vi "login.vi"(8 "error in (no error)":errorcluster, 10 "element":string, 11 "Masterv2 in":refnum<class "Masterv2.lvclass">) -> (0 "error out":errorcluster, 2 "x >= 0?":bool, 3 "Masterv2 out":refnum<class "Masterv2.lvclass">)   [LabVIEW 2014, in "Main Libraryv2.lvlib" / "Masterv2.lvclass"]
uses:
  Master/Masterv2.lvclass
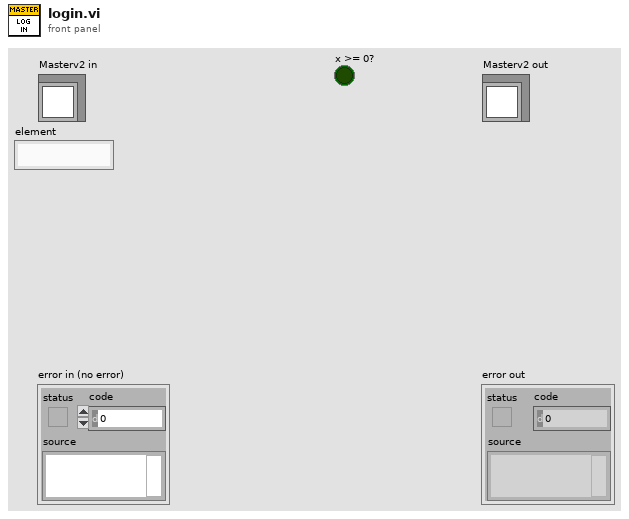
[diagram p1: front panel]
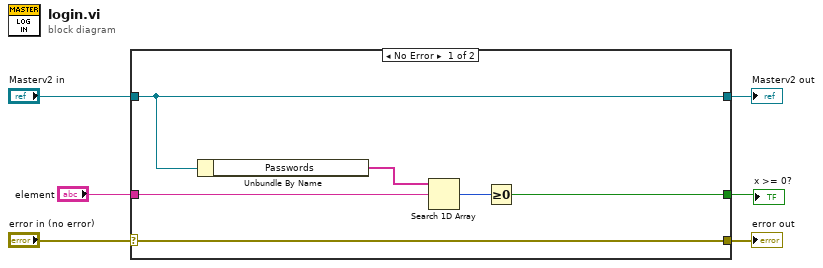
[diagram p0: block diagram]
diagram:
  n1 = case shown="No Error" "error in (no error)" {
    selector: "error in (no error)" -> [w7 w14]
    tunnel: [w7 w14] -> w5
    tunnel: [w8 w13] -> w3
    tunnel: "Masterv2 in" -> [w8 w13]
    tunnel: [w10 _] -> w2
    tunnel: "element" -> [w9 _]
    frame No Error {
      n2 = Unbundle By Name(w8) -> ("Passwords"=w12:string[])
      n3 = Search 1D Array(1D array=w12, element=w9) -> (index of element=w11:i32)  [unwired: 1 in]
      n4 = Greater Or Equal To 0?(x=w11) -> (x >= 0?=w10:bool)
    }
    frame Error {
    }
  }
  "error out" <- w5
  "Masterv2 out" <- w3
  "x >= 0?" <- w2
